vi "Create Doodle and background.vi"(10 "Doodle in":path=path "\\\\vmware-host\\Shared Folders/Downloads/Game/Game/monito1.png", 11 "Background":path=path "\\\\vmware-host\\Shared Folders/Downloads/Game/Game/background.png") -> (1 "top":i16, 2 "Doodle out":T1, 3 "background":picture, 4 "bottom":i16)   [LabVIEW 2019]
uses:
  <vilib>/picture/picture.llb/imagedata.ctl
panel:
  out "new picture":picture
  out "Init Data Out":u16[](array[numeric]) format="%.0x"
  out "back":u16[](array[numeric]) format="%.0x"
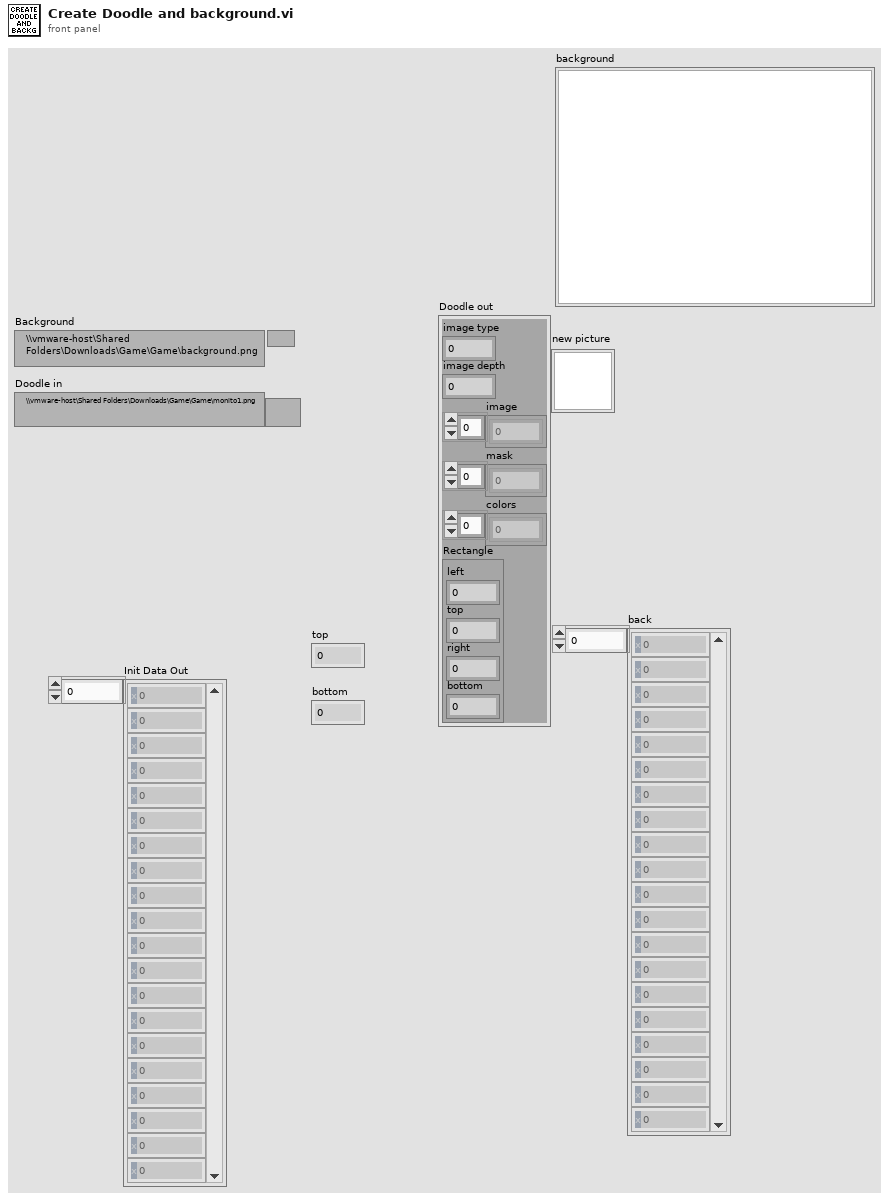
[diagram p1: front panel]
types:
  T1 = typedef "imagedata.ctl" = cluster{"image type":i32, "image depth":i32, "image":u8[], "mask":u8[], "colors":u32[], "Rectangle":cluster{"left":i16, "top":i16, "right":i16, "bottom":i16}}
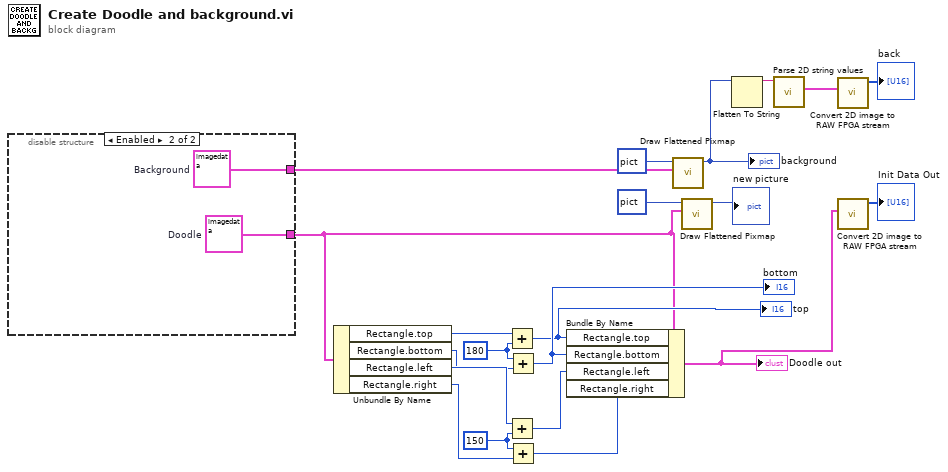
[diagram p0: block diagram]
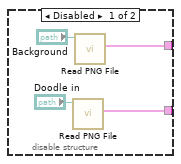
[diagram p2: hidden frame]
diagram:
  w16 = i16 150 ("y")
  w14 = i16 180 ("y")
  n1 = disable-structure shown="Enabled" {
    disable-tunnel: [w23 w27] -> w21
    disable-tunnel: [w22 w26] -> w2
    frame Disabled {
      n2 = call <vilib>:"Read PNG File.vi"("path to PNG file"="Doodle in") -> ("image data"=w22:T1)  [unwired: 8 in, 2 out]
      n3 = call <vilib>:"Read PNG File.vi"("path to PNG file"="Background") -> ("image data"=w23:T1)  [unwired: 8 in, 2 out]
    }
    frame Enabled {
      w26 = T1 {"image type"=0, "image depth"=24, "image"=array[9408 elements], "mask"=[0, 15, 254, 0, 0, 0, 0, 0, 0, 63, 255, 128, 0, 0, 0, 0, 0, 127, 255, 224, 0, 0, 0, 0, 0, 255, 255, 240, 0, 0, 0, 0, 3, 255, 255, 248, 0, 0, 0, 0, 7, 255, 255, 254, 0, 0, 0, 0, 15, 255, 255, 254, 0, 0, 0, 0, 31, 255, 255, 255, 0, 0, 0, 0, 63, 255, 255, 255, 128, 0, 0, 0, 63, 255, 255, 255, 192, 0, 0, 0, 127, 255, 255, 255, 192, 0, 0, 0, 127, 255, 255, 255, 224, 0, 0, 0, 255, 255, 255, 255, 224, 0, 0, 0, 255, 255, 255, 255, 240, 0, 0, 0, 255, 255, 255, 255, 240, 0, 0, 0, 255, 255, 255, 255, 248, 0, 0, 0, 255, 255, 255, 255, 252, 0, 24, 0, 255, 255, 255, 255, 254, 0, 62, 0, 255, 255, 255, 255, 255, 247, 254, 0, 255, 255, 255, 255, 255, 255, 255, 0, 255, 255, 255, 255, 255, 255, 255, 0, 255, 255, 255, 255, 255, 255, 255, 0, 255, 255, 255, 255, 255, 255, 255, 0, 255, 255, 255, 255, 255, 255, 255, 0, 255, 255, 255, 255, 255, 255, 255, 0, 255, 255, 255, 255, 255, 255, 255, 0, 255, 255, 255, 255, 255, 255, 255, 0, 255, 255, 255, 255, 252, 0, 127, 0, 255, 255, 255, 255, 248, 0, 63, 0, 255, 255, 255, 255, 240, 0, 30, 0, 255, 255, 255, 255, 240, 0, 4, 0, 255, 255, 255, 255, 240, 0, 0, 0, 255, 255, 255, 255, 240, 0, 0, 0, 255, 255, 255, 255, 240, 0, 0, 0, 255, 255, 255, 255, 240, 0, 0, 0, 255, 255, 255, 255, 240, 0, 0, 0, 255, 255, 255, 255, 240, 0, 0, 0, 255, 255, 255, 255, 240, 0, 0, 0, 255, 255, 255, 255, 240, 0, 0, 0, 255, 255, 255, 255, 240, 0, 0, 0, 255, 255, 255, 255, 240, 0, 0, 0, 255, 255, 255, 255, 248, 0, 0, 0, 255, 255, 255, 255, 248, 0, 0, 0, 127, 255, 255, 255, 248, 0, 0, 0, 127, 255, 255, 255, 248, 0, 0, 0, 127, 255, 255, 255, 248, 0, 0, 0, 127, 255, 255, 255, 240, 0, 0, 0, 127, 255, 255, 255, 128, 0, 0, 0, 31, 255, 15, 7, 128, 0, 0, 0, 7, 15, 15, 7, 128, 0, 0, 0, 7, 15, 15, 7, 0, 0, 0, 0, 7, 14, 15, 7, 248, 0, 0, 0, 15, 15, 15, 231, 248, 0, 0, 0, 15, 239, 239, 231, 240, 0, 0, 0, 7, 239, 231, 224, 0, 0, 0, 0, 7, 231, 224, 128, 0, 0, 0, 0], "colors"=[], "Rectangle"={"left"=0, "top"=0, "right"=56, "bottom"=56}}  # Doodle
      w27 = T1 {"image type"=0, "image depth"=24, "image"=array[230400 elements], "mask"=array[9600 elements], "colors"=[], "Rectangle"={"left"=0, "top"=0, "right"=320, "bottom"=240}}  # Background
    }
  }
  n4 = Unbundle By Name(w2) -> ("Rectangle.top"=w10:i16, "Rectangle.bottom"=w15:i16, "Rectangle.left"=w17:i16, "Rectangle.right"=w19:i16)
  n5 = Add(x=w10, y=w14) -> (x+y=w11:i16)
  "top" <- w11
  n6 = Add(x=w17, y=w16) -> (x+y=w18:i16)
  n7 = Add(x=w14, y=w15) -> (x+y=w12:i16)
  "bottom" <- w12
  n8 = Add(x=w16, y=w19) -> (x+y=w20:i16)
  n9 = Bundle By Name(cluster=w2, "Rectangle.top"=w11, "Rectangle.bottom"=w12, "Rectangle.left"=w18, "Rectangle.right"=w20) -> (w4:T1)
  "Doodle out" <- w4
  n10 = call <vilib>:"Draw Flattened Pixmap.vi"("image data"=w21, "picture"=picture data[5B]) -> ("new picture"=w8:picture)  [unwired: 7 in]
  "background" <- w8
  n11 = call <vilib>:"Draw Flattened Pixmap.vi"("image data"=w2, "picture"=picture data[5B]) -> ("new picture"=→"new picture":picture)  [unwired: 7 in]
  n12 = Flatten To String(anything=w8) -> (data string=w9:string)  [unwired: 3 in, 2 out]
  n13 = call "Parse 2D string values.vi"("data string in"=w9) -> ("image data"=w7:T1)  [unwired: 8 in, 2 out]
  n14 = call "Convert 2D image to RAW FPGA stream.vi"("image data"=w7) -> ("data"=→"back":u16[])  [unwired: 9 in, 1 out]
  n15 = call "Convert 2D image to RAW FPGA stream.vi"("image data"=w4) -> ("data"=→"Init Data Out":u16[])  [unwired: 9 in, 1 out]
